vi "BWR_Simulator.vi"() -> ()   [LabVIEW 2021]
uses:
  <vilib>/numeric/Random Number (Range) DBL.vi
  <vilib>/Utility/file.llb/Read Delimited Spreadsheet (I64).vi
panel:
  out "Slide 4":dbl(slide)=110.0 scale=0.0..110.0
  out "Slide 3":dbl(slide)=110.0 scale=0.0..110.0
  out "Slide 2":dbl(slide)=110.0 scale=0.0..110.0
  out "Slide":dbl(slide)=110.0 scale=0.0..110.0
  in  "Tab Control":enum32{"Page 1", "Page 2"}(tab)
  out "Reactor Power\n(MWth)":i64
  out "Core Outlet Temp\n(C)":i64
  out "Core Inlet Temp\n(C)":i64
  out "Core Outlet Pressure\n(kPa)":i64
  out "Coolant Flow Rate\n(kg/s)":i64
  out "Electric Output":dbl(graph)
  out "Reactor Power":dbl(graph)
  out "Electric Output\n(MWe)":i64
  out "Core Inlet Temp":dbl(graph)
  out "Core Outlet Temp":dbl(graph)
  out "Core Outlet Pressure":dbl(graph)
  out "Coolant Flow Rate":dbl(graph)
  out "Feedwater Temperature":dbl(graph)
  out "Feedwater Temperature\n(C)":dbl
  out "Feedwater Flow":dbl(graph)
  out "Feedwater Flow\n(kg/s)":dbl
  out "Steam Temperature":dbl(graph)
  out "Steam Temperature\n(C)":dbl
  out "Steam Pressure":dbl(graph)
  out "Steam Pressure\n(kPa)":dbl
  out "Steam Flow":dbl(graph)
  out "Steam Flow\n(kg/s)":i64
  out "Control Rods Positon\n(% Inserted)":i64
  out "% Full Power Meter":dbl(knob)=10.0 scale=10.0..110.0
  in  "% Full Power\nControl":i32(slide)=10 min=10 max=110 step=10 scale=10.0..110.0
  in  "Stop Simulation":bool
  # "Control Rods"
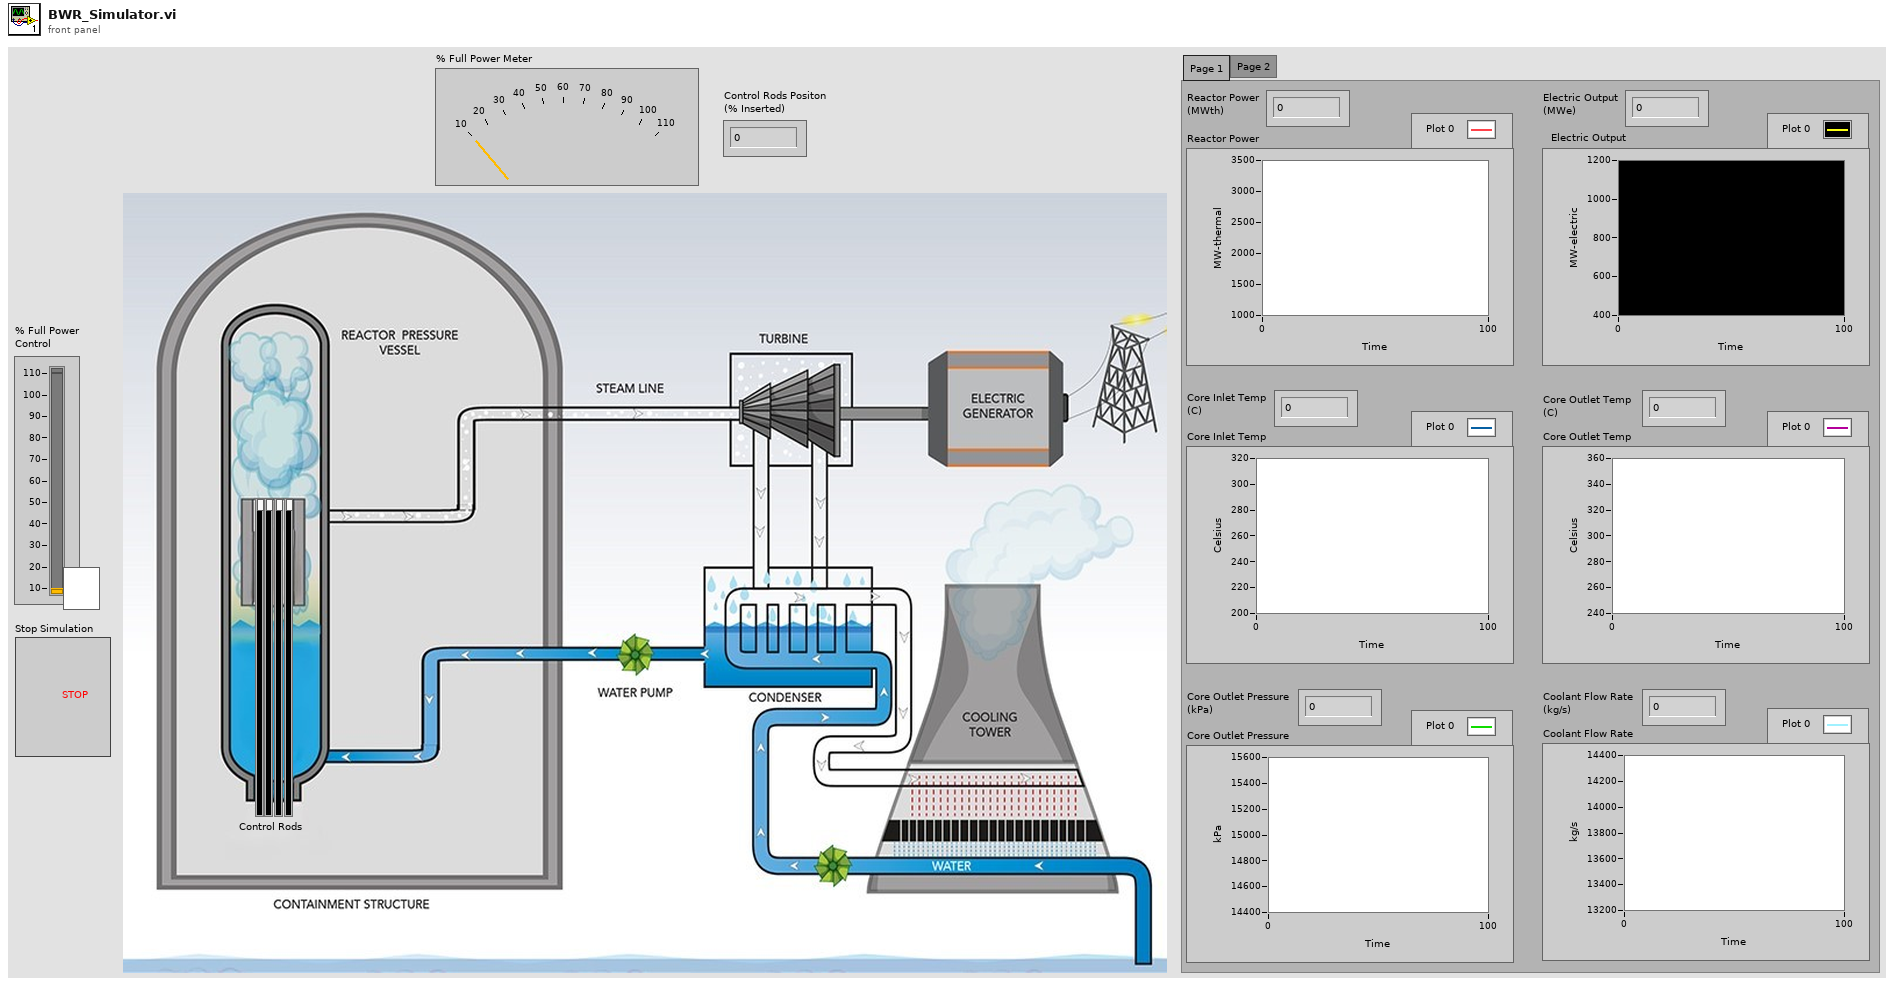
[diagram p1: front panel]
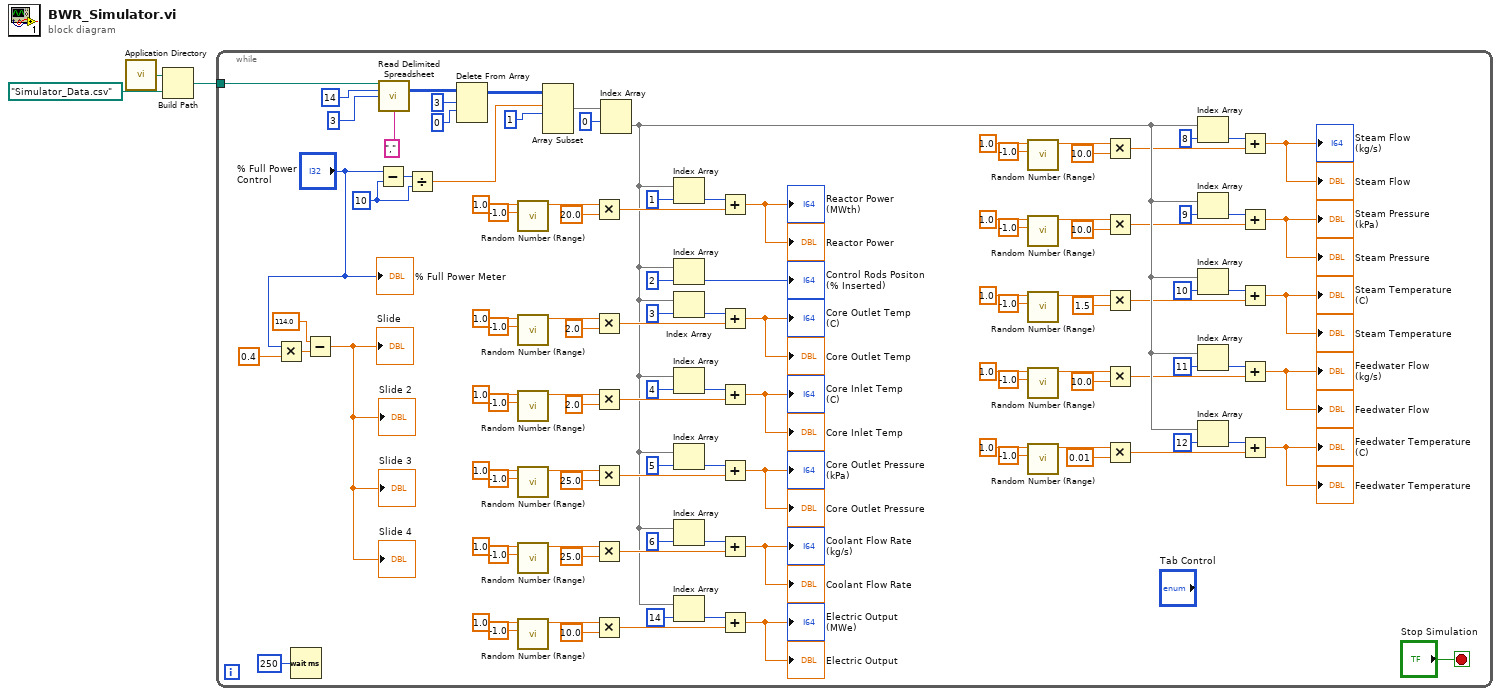
[diagram p0: block diagram]
diagram:
  n1 = call <vilib>:"Application Directory.vi"() -> ("Application Directory"=w3:path)
  n2 = Build Path(base path=w3, name or relative path=path "Simulator_Data.csv") -> (appended path=w1:path)
  n3 = while {
    tunnel: w1 -> [w115]
    stop <- "Stop Simulation" stop-if-true
    w103 = 10 ("y")
    n4 = Multiply(x="% Full Power\nControl", y=0.4) -> (x*y=w6:dbl)
    n5 = Wait (ms)(milliseconds to wait=u32 250) -> ()  [unwired: 1 out]
    n6 = Subtract(x=114.0, y=w6) -> (x-y=→"Slide" →"Slide 3" →"Slide 4" →"Slide 2":dbl)
    n7 = Subtract(x="% Full Power\nControl", y=w103) -> (x-y=w104:i32)
    n8 = call-poly <vilib>:"Read Delimited Spreadsheet.vi"("file path (dialog if empty)"=w115, "number of rows (all:-1)"=14, "start of read offset (chars.:0)"=3, "delimiter (\\t)"="," ("delimiter (\\t)")) -> ("all rows"=w109:i64[][])  [unwired: 6 in, 5 out]
    n9 = Divide(x=w104, y=w103) -> (x/y=w105:dbl)
    n10 = Delete From Array(array=w109, length=3, index (row)=0) -> (array with subset deleted=w106:i64[][])  [unwired: 1 in, 1 out]
    n11 = call-poly <vilib>:"Random Number (Range).vi"("lower bound (0)"=-1.0, "upper bound (100)"=1.0) -> ("number"=w75:dbl)  [unwired: 9 in]
    n12 = call-poly <vilib>:"Random Number (Range).vi"("lower bound (0)"=-1.0, "upper bound (100)"=1.0) -> ("number"=w66:dbl)  [unwired: 9 in]
    n13 = call-poly <vilib>:"Random Number (Range).vi"("lower bound (0)"=-1.0, "upper bound (100)"=1.0) -> ("number"=w62:dbl)  [unwired: 9 in]
    n14 = call-poly <vilib>:"Random Number (Range).vi"("lower bound (0)"=-1.0, "upper bound (100)"=1.0) -> ("number"=w58:dbl)  [unwired: 9 in]
    n15 = call-poly <vilib>:"Random Number (Range).vi"("lower bound (0)"=-1.0, "upper bound (100)"=1.0) -> ("number"=w53:dbl)  [unwired: 9 in]
    n16 = call-poly <vilib>:"Random Number (Range).vi"("lower bound (0)"=-1.0, "upper bound (100)"=1.0) -> ("number"=w50:dbl)  [unwired: 9 in]
    n17 = Array Subset(array=w106, index (row)=w105, length (row)=1 ("length")) -> (w102:i64[][])  [unwired: 2 in]
    n18 = Multiply(x=w75, y=20.0) -> (x*y=w87:dbl)
    n19 = Multiply(x=w66, y=2.0) -> (x*y=w78:dbl)
    n20 = Multiply(x=w62, y=2.0) -> (x*y=w61:dbl)
    n21 = Multiply(x=w58, y=25.0) -> (x*y=w70:dbl)
    n22 = Multiply(x=w53, y=25.0) -> (x*y=w56:dbl)
    n23 = Multiply(x=w50, y=10.0) -> (x*y=w83:dbl)
    n24 = Index Array(array=w102, index (row)=0) -> (element=w45:i64[])  [unwired: 1 in]
    n25 = Index Array(array=w45, index=1) -> (element=w88:i64)
    n26 = Index Array(array=w45, index=2) -> (element=→"Control Rods Positon\n(% Inserted)":i64)
    n27 = Index Array(array=w45, index=3) -> (element=w81:i64)
    n28 = Index Array(array=w45, index=4) -> (element=w79:i64)
    n29 = Index Array(array=w45, index=5) -> (element=w73:i64)
    n30 = Index Array(array=w45, index=6) -> (element=w71:i64)
    n31 = Index Array(array=w45, index=14) -> (element=w84:i64)
    n32 = Add(x=w88, y=w87) -> (x+y=→"Reactor Power\n(MWth)" →"Reactor Power":dbl)
    n33 = Add(x=w81, y=w78) -> (x+y=→"Core Outlet Temp\n(C)" →"Core Outlet Temp":dbl)
    n34 = Add(x=w79, y=w61) -> (x+y=→"Core Inlet Temp\n(C)" →"Core Inlet Temp":dbl)
    n35 = Add(x=w73, y=w70) -> (x+y=→"Core Outlet Pressure\n(kPa)" →"Core Outlet Pressure":dbl)
    n36 = Add(x=w71, y=w56) -> (x+y=→"Coolant Flow Rate\n(kg/s)" →"Coolant Flow Rate":dbl)
    n37 = Add(x=w84, y=w83) -> (x+y=→"Electric Output" →"Electric Output\n(MWe)":dbl)
    n38 = call-poly <vilib>:"Random Number (Range).vi"("lower bound (0)"=-1.0, "upper bound (100)"=1.0) -> ("number"=w41:dbl)  [unwired: 9 in]
    n39 = call-poly <vilib>:"Random Number (Range).vi"("lower bound (0)"=-1.0, "upper bound (100)"=1.0) -> ("number"=w34:dbl)  [unwired: 9 in]
    n40 = call-poly <vilib>:"Random Number (Range).vi"("lower bound (0)"=-1.0, "upper bound (100)"=1.0) -> ("number"=w27:dbl)  [unwired: 9 in]
    n41 = call-poly <vilib>:"Random Number (Range).vi"("lower bound (0)"=-1.0, "upper bound (100)"=1.0) -> ("number"=w13:dbl)  [unwired: 9 in]
    n42 = call-poly <vilib>:"Random Number (Range).vi"("lower bound (0)"=-1.0, "upper bound (100)"=1.0) -> ("number"=w20:dbl)  [unwired: 9 in]
    n43 = Multiply(x=w41, y=10.0) -> (x*y=w39:dbl)
    n44 = Multiply(x=w34, y=10.0) -> (x*y=w31:dbl)
    n45 = Multiply(x=w27, y=1.5) -> (x*y=w23:dbl)
    n46 = Multiply(x=w13, y=10.0) -> (x*y=w9:dbl)
    n47 = Multiply(x=w20, y=0.01) -> (x*y=w17:dbl)
    n48 = Index Array(array=w45, index=8) -> (element=w38:i64)
    n49 = Index Array(array=w45, index=9) -> (element=w32:i64)
    n50 = Index Array(array=w45, index=10) -> (element=w25:i64)
    n51 = Index Array(array=w45, index=11) -> (element=w11:i64)
    n52 = Index Array(array=w45, index=12) -> (element=w18:i64)
    n53 = Add(x=w38, y=w39) -> (x+y=→"Steam Flow\n(kg/s)" →"Steam Flow":dbl)
    n54 = Add(x=w32, y=w31) -> (x+y=→"Steam Pressure\n(kPa)" →"Steam Pressure":dbl)
    n55 = Add(x=w25, y=w23) -> (x+y=→"Steam Temperature\n(C)" →"Steam Temperature":dbl)
    n56 = Add(x=w11, y=w9) -> (x+y=→"Feedwater Flow\n(kg/s)" →"Feedwater Flow":dbl)
    n57 = Add(x=w18, y=w17) -> (x+y=→"Feedwater Temperature\n(C)" →"Feedwater Temperature":dbl)
    "% Full Power Meter" <- "% Full Power\nControl"
  }
